vi "Shooter Logic Test.vi"() -> ()   [LabVIEW 2013]
uses:
  <vilib>/Rock Robotics/WPI/Solenoid/WPI_SolenoidValue.ctl
  Robot Code/Shooter/Shooter Manual Control.ctl
  Robot Code/Shooter/Shooter Command.ctl
  Common Code/Shooter State.ctl
panel:
  out "State":T1
  in  "Shooter Control":T2
  out "Trigger":bool
  out "Release":bool
  out "Add":bool
  in  "stop":bool
  out "Trigger":T4
  out "Release":T4
  out "Add":T4
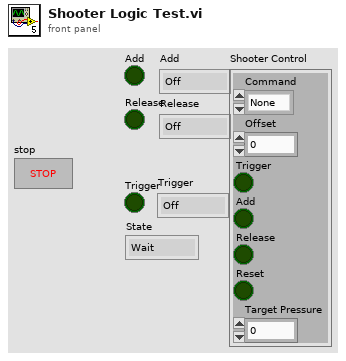
[diagram p1: front panel]
types:
  T1 = typedef "Shooter State.ctl" = enum16{"Wait", "Fill Piston", "Trigger", "Reset"}
  T2 = typedef "Shooter Manual Control.ctl" = cluster{"Command":T3, "Offset":dbl, "Trigger":bool, "Add":bool, "Release":bool, "Reset":bool, "Target Pressure":dbl}
  T3 = typedef "Shooter Command.ctl" = enum16{"None", "Warmup", "Shoot"}
  T4 = typedef "WPI_SolenoidValue.ctl" = enum16{"Off", "On", "Forward", "Reverse"}
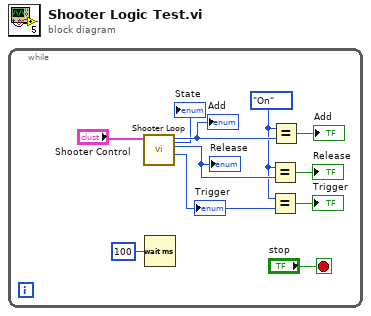
[diagram p0: block diagram]
diagram:
  n1 = while {
    stop <- "stop" stop-if-true
    w7 = WPI_SolenoidValue."On" ("y")
    n2 = call "Shooter Loop.vi"("Shooter Control"="Shooter Control") -> ("Trigger"=w6:T4, "Release"=w8:T4, "Add"=w9:T4, "State"=→"State":T1)  [unwired: 7 in]
    "Add" <- w9
    "Release" <- w8
    "Trigger" <- w6
    n3 = Wait (ms)(milliseconds to wait=u32 100) -> ()  [unwired: 1 out]
    n4 = Equal?(x=w7, y=w8) -> (x = y?=→"Release":bool)
    n5 = Equal?(x=w7, y=w6) -> (x = y?=→"Trigger":bool)
    n6 = Equal?(x=w7, y=w9) -> (x = y?=→"Add":bool)
  }
